vi "Playback.vi"() -> ()   [LabVIEW 2012]
doc: "This VI reads records of data from the logging table in the LabVIEW.mdb database. \n\nAll the records from the table are retrieved at one time using the DB Tools Select Data VI. This data is in the format of a two dimensional array of variants. This array is indexed and each of the values are converted back to their original data types."
uses:
  Connection.llb/DB Tools Open Connec (Path).vi
  NI_Database_API_64.lvlib
  _DB Variant To Data/Database Variant To Data.xnode
panel:
  out "Core Measuments":dbl[][](graph)
  out "record number":i32
  in  "previous record":bool
  in  "next record":bool
  in  "stop":bool
  out "min temperature value":dbl format="%.2f"
  out "max temperature value":dbl format="%.2f"
  out "min pressure value":dbl format="%.2f"
  out "max pressure value":dbl format="%.2f"
  out "Core Temperature":dbl[](graph)
  out "Core Pressure":dbl[](graph)
  # "INSTRUCTIONS:\n\nRun the VI to retrieve data from a table written by the Logging Example VI.\nOnce the VI begins, it displays the 0th (zeroth) record in the table. You can navigate the recordset using the previous record and next record buttons."
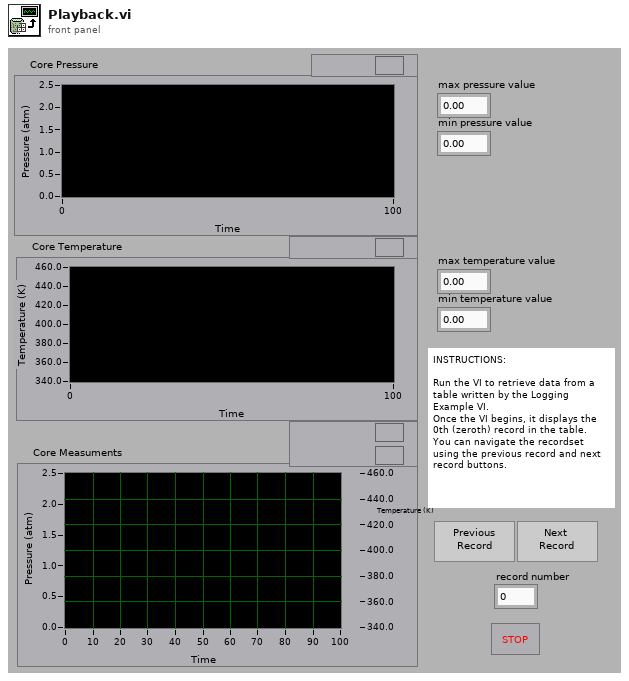
[diagram p1: front panel]
types:
  T1 = typedef "NI_Database_API_64.lvlib/Conn ObjectReference.ctl" = refnum<k1>
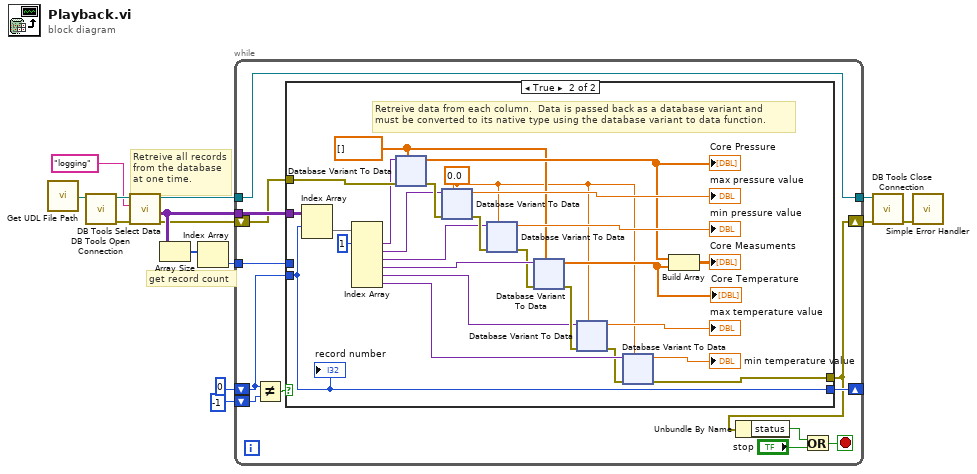
[diagram p0: block diagram]
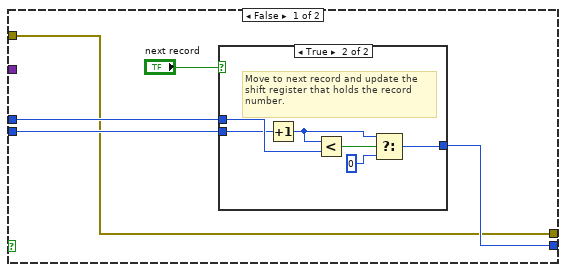
[diagram p2: hidden frame]
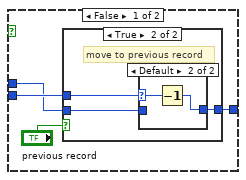
[diagram p3: hidden frame]
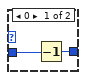
[diagram p5: hidden frame]
diagram:
  # "Retreive all records\nfrom the database\nat one time."
  # "get record count"
  n1 = call "Get UDL File Path.vi"() -> ("UDL file path"=w1:path)  [unwired: 1 in]
  n2 = call-poly "DB Tools Open Connection.vi"("connection information"=w1) -> ("error out"=w14:errorcluster, "connection reference"=w13:T1)  [unwired: 7 in]
  n3 = call "DB Tools Select Data.vi"("error in (no error)"=w14, "table"="logging", "connection reference"=w13) -> ("error out"=w5:errorcluster, "data"=w10:variant[][], "connection reference out"=w11:T1)  [unwired: 3 in]
  n4 = Array Size(array=w10) -> (size(s)=w7:i32[])
  n5 = Index Array(array=w7) -> (element=w6:i32)  [unwired: 1 in]
  n6 = while {
    tunnel: w11 -> [w15]
    tunnel: w10 -> [w21]
    shift-right: [w23] -> _
    shift-left: 0 -> [w24]
    shift-left: -1 -> [w26]
    tunnel: w6 -> [w22]
    shift-right: [w19] -> w4
    shift-left: w5 -> [w20]
    tunnel: [w15] -> w2
    stop <- w18 stop-if-true
    n7 = Not Equal?(x=w24, y=w26) -> (x != y?=w25:bool)
    n8 = case shown="True" w25 {
      tunnel: w24 -> [w30 w68]
      tunnel: [w29 w68] -> w23
      tunnel: w22 -> [w28 _]
      tunnel: w21 -> [_ w66]
      tunnel: w20 -> [w27 w65]
      tunnel: [w27 w62] -> w19
      frame False {
        n9 = case shown="True" "next record" {
          tunnel: w30 -> [w34 w45]
          tunnel: [w33 w47] -> w29
          tunnel: w28 -> [w32 w49]
          frame False {
            n10 = case shown="True" "previous record" {
              tunnel: w34 -> [w36 w38]
              tunnel: [w36 w39] -> w33
              tunnel: w32 -> [_ w37]
              frame False {
              }
              frame True {
                # "move to previous record"
                n11 = case shown="Default" w38 {
                  selector: w38 -> [_ w42]
                  tunnel: [w41 w43] -> w39
                  tunnel: w37 -> [w40 _]
                  frame 0 {
                    n12 = Decrement(x=w40) -> (x-1=w41:i32)
                  }
                  frame Default {
                    n13 = Decrement(x=w42) -> (x-1=w43:i32)
                  }
                }
              }
            }
          }
          frame True {
            # "Move to next record and update the \nshift register that holds the record \nnumber."
            n14 = Increment(x=w45) -> (x+1=w46:i32)
            n15 = Less?(x=w46, y=w49) -> (x < y?=w48:bool)
            n16 = Select(t=w46, s=w48, f=0) -> (s? t:f=w47:i32)
          }
        }
      }
      frame True {
        w50 = 0.0
        w51 = dbl[] [] ("Array Constant")
        # "Retreive data from each column.  Data is passed back as a database variant and \nmust be converted to its native type using the database variant to data function."
        n17 = Index Array(array=w66, index (row)=w68) -> (element=w75:variant[])  [unwired: 1 in]
        n18 = Index Array(array=w75, index #1=1 ("Index")) -> (element #1=w59:variant, element #2=w58:variant, element #3=w57:variant, element #4=w56:variant, element #5=w55:variant, element #6=w54:variant)  [unwired: 5 in]
        n19 = xnode "Database Variant To Data"("database variant"=w59, "error in"=w65, "type"=w51) -> ("data"=w69:dbl[], "error out"=w61:errorcluster)
        "Core Pressure" <- w69
        n20 = xnode "Database Variant To Data"("database variant"=w58, "error in"=w61, "type"=w50) -> ("data"=→"max pressure value":dbl, "error out"=w64:errorcluster)
        n21 = xnode "Database Variant To Data"("database variant"=w57, "error in"=w64, "type"=w50) -> ("data"=→"min pressure value":dbl, "error out"=w53:errorcluster)
        n22 = xnode "Database Variant To Data"("database variant"=w56, "error in"=w53, "type"=w51) -> ("data"=w72:dbl[], "error out"=w63:errorcluster)
        "Core Temperature" <- w72
        n23 = xnode "Database Variant To Data"("database variant"=w55, "error in"=w63, "type"=w50) -> ("data"=→"max temperature value":dbl, "error out"=w52:errorcluster)
        n24 = xnode "Database Variant To Data"("database variant"=w54, "error in"=w52, "type"=w50) -> ("data"=→"min temperature value":dbl, "error out"=w62:errorcluster)
        n25 = Build Array(w69, w72) -> (→"Core Measuments":dbl[][])
        "record number" <- w68
      }
    }
    n26 = Unbundle By Name(w19) -> ("status"=w16:bool)
    n27 = Or(x=w16, y="stop") -> (x .or. y?=w18:bool)
  }
  n28 = call "DB Tools Close Connection.vi"("error in (no error)"=w4, "connection reference"=w2) -> ("error out"=w3:errorcluster)  [unwired: 5 in]
  n29 = call <vilib>:"Simple Error Handler.vi"("error in (no error)"=w3) -> ()  [unwired: 4 in, 5 out]
